vi "Validate Start Stop Positions.vi"(8 "error in (no error)":errorcluster, 11 "Video File in":refnum<class "Video File.lvclass">) -> (0 "error out":errorcluster, 3 "Video File out":refnum<class "Video File.lvclass">)   [LabVIEW 2018, in "Video File.lvclass"]
uses:
  Video File.lvclass
  Video File.lvclass/Video File.ctl
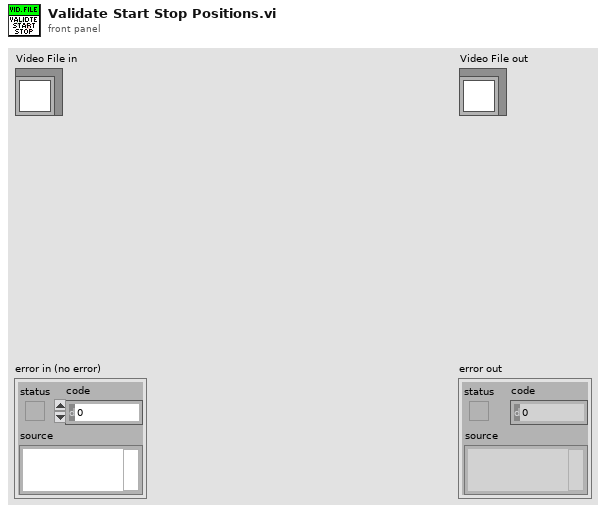
[diagram p1: front panel]
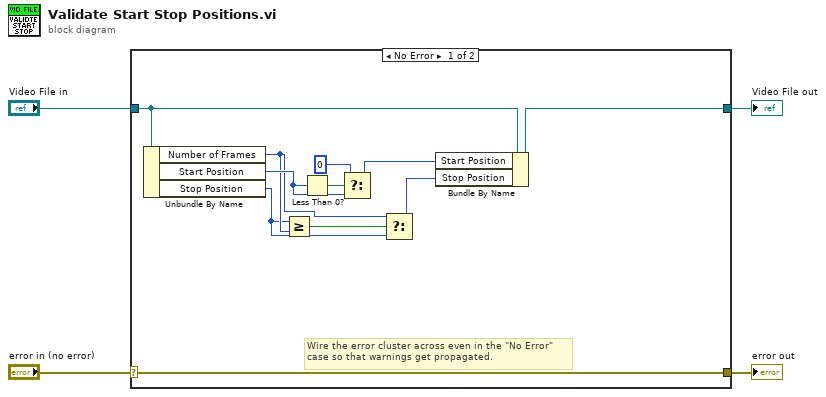
[diagram p0: block diagram]
diagram:
  n1 = case shown="No Error" "error in (no error)" {
    selector: "error in (no error)" -> [w15 w17]
    tunnel: [w15 w17] -> w3
    tunnel: [w13 w16] -> w1
    tunnel: "Video File in" -> [w14 w16]
    frame No Error {
      # "Wire the error cluster across even in the \"No Error\"\ncase so that warnings get propagated."
      n2 = Unbundle By Name(w14) -> ("Number of Frames"=w7:u32, "Start Position"=w11:u32, "Stop Position"=w6:u32)
      n3 = Greater Or Equal?(x=w6, y=w7) -> (x >= y?=w8:bool)
      n4 = Less Than 0?(x=w11) -> (x < 0?=w12:bool)
      n5 = Select(t=u32 0, s=w12, f=w11) -> (s? t:f=w9:u32)
      n6 = Select(t=w7, s=w8, f=w6) -> (s? t:f=w5:u32)
      n7 = Bundle By Name(cluster=w14, "Start Position"=w9, "Stop Position"=w5) -> (w13:refnum<class "Video File.lvclass">)
    }
    frame Error {
    }
  }
  "error out" <- w3
  "Video File out" <- w1
